vi "Periodic Tasks.vi"(8 "error out":errorcluster) -> ()   [LabVIEW 2011]
doc: "This VI runs in parallel to other tasks. It can contain as many user-defined periodic loops as you need. These can carry out PID or other sorts of timed response."
uses:
  <vilib>/Rock Robotics/WPI/Camera/WPI_CameraFrameRate.ctl
  <vilib>/Rock Robotics/WPI/Camera/WPI_CameraImageSize.ctl
  <vilib>/Rock Robotics/SystemInterfaces/DIO/FPGA_DIOChannel.ctl
  <vilib>/Rock Robotics/SystemInterfaces/Typedef/FPGA_TypedefDigitalModule.ctl
  <vilib>/Rock Robotics/WPI/Relay/WPI_RelayValue.ctl
  <vilib>/Rock Robotics/WPI/Counter/WPI_CounterDigitalInputToDigitalSource.vi
  Robot Global Data.vi
panel:
  out "Lights?":bool
  in  "Density Threshold":dbl=3.0
  in  "Dense Adjustment Factor":dbl=0.89
  out "Pressure":dbl
  out "Integral":dbl
  out "Error":dbl
  out "Waveform Chart":dynamicdata(graph)
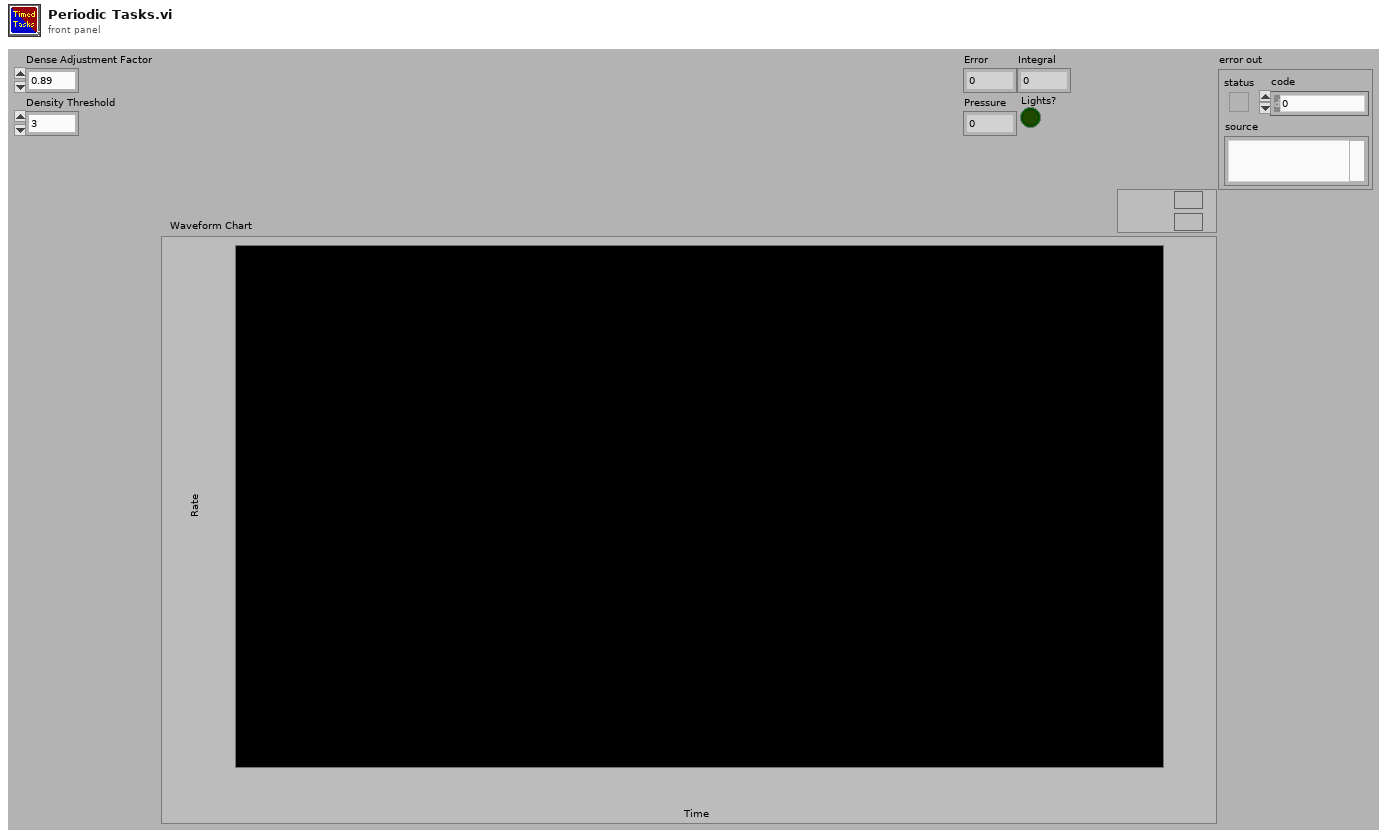
[diagram p1: front panel]
types:
  T1 = typedef "FPGA_DIOChannel.ctl" = enum8{"DIO 1", "DIO 2", "DIO 3", "DIO 4", "DIO 5", "DIO 6", "DIO 7", "DIO 8", "DIO 9", "DIO 10", "DIO 11", "DIO 12", "DIO 13", "DIO 14", "Invalid"}
  T2 = typedef "FPGA_TypedefDigitalModule.ctl" = enum16{"Digital Module 1", "Digital Module 2"}
  T3 = typedef "WPI_CameraImageSize.ctl" = enum16{"640x480", "320x240", "160x120"}
  T4 = typedef "WPI_CameraFrameRate.ctl" = u32
  T5 = typedef "WPI_JoystickDevRef.ctl" = cluster{"Device":T6}
  T6 = typedef "WPI_JoystickDeviceEnum.ctl" = enum16{"USB 1", "USB 2", "USB 3", "USB 4", "Kinect 1", "Kinect 2"}
  T7 = typedef "WPI_JoystickButtonState.ctl" = cluster{"Button 1":bool, "Button 2":bool, "Button 3":bool, "Button 4":bool, "Button 5":bool, "Button 6":bool, "Button 7":bool, "Button 8":bool, "Button 9":bool, "Button 10":bool, "Button 11":bool, "Button 12":bool}
  T8 = typedef "WPI_CameraDevRef.ctl" = cluster{"Camera Address":string, "CameraStatus":errorcluster, "Acquire Image Notifier":refnum<notifier>}
  T9 = typedef "WPI_AnalogChannelDevRef.ctl" = cluster{"DevStatus":errorcluster, "Analog Module":T10, "Analog Channel":T11}
  T10 = typedef "FPGA_TypedefAnalogModule.ctl" = enum16{"Analog Module 1", "Analog Module 2"}
  T11 = typedef "FPGA_AIChannel.ctl" = enum8{"AI 1", "AI 2", "AI 3", "AI 4", "AI 5", "AI 6", "AI 7", "AI 8", "Invalid"}
  T12 = typedef "WPI_RelayValue.ctl" = enum16{"Off", "On", "Forward", "Reverse"}
  T13 = typedef "WPI_RelayDevRef.ctl" = cluster{"DevStatus":errorcluster, "Relay Channel":T14, "Digital Module":T2, "Relay Direction":T15}
  T14 = typedef "FPGA_DIORelayChannel.ctl" = enum8{"Relay 1", "Relay 2", "Relay 3", "Relay 4", "Relay 5", "Relay 6", "Relay 7", "Relay 8", "Invalid"}
  T15 = typedef "WPI_RelayDirection.ctl" = enum16{"Both directions", "Forward only", "Reverse only"}
  T16 = typedef "WPI_DigitalInputDevRef.ctl" = cluster{"DevStatus":errorcluster, "DIO Channel":T1, "Digital Module":T2}
  T17 = typedef "FPGA_CounterEncoderSourceConvertionLVSourceType.ctl" = cluster{"DevStatus":errorcluster, "AnalogTriggerMode?":bool, "DigitalMode":cluster{"Digital Module":T2, "DIO Channel":T18}, "AnalogTriggerMode":cluster{"AnalogTriggerIndex":T19, "OutputType":T20}}
  T18 = typedef "FPGA_DIODigitalSourceChannel.ctl" = enum8{"DIO 1", "DIO 2", "DIO 3", "DIO 4", "DIO 5", "DIO 6", "DIO 7", "DIO 8", "DIO 9", "DIO 10", "DIO 11", "DIO 12", "DIO 13", "DIO 14", "Disabled"}
  T19 = typedef "FPGA_AnalogTriggerIndex.ctl" = enum8{"Trig 0", "Trig 1", "Trig 2", "Trig 3", "Trig 4", "Trig 5", "Trig 6", "Trig 7", "Invalid"}
  T20 = typedef "FPGA_AnalogTriggerOutType.ctl" = enum16{"InWindow", "TriggerState", "Rising", "Falling"}
  T21 = typedef "WPI_EncoderDevRef.ctl" = cluster{"DevStatus":errorcluster, "EncoderIndex":T22, "CounterIndex":T23, "DistancePerCount":dbl, "Decoding Type":T24}
  T22 = typedef "FPGA_EncoderIdx.ctl" = enum8{"Enc 0", "Enc 1", "Enc 2", "Enc 3", "Invalid"}
  T23 = typedef "FPGA_CounterCtrSystemIndex.ctl" = enum8{"Ctr 0", "Ctr 1", "Ctr 2", "Ctr 3", "Ctr 4", "Ctr 5", "Ctr 6", "Ctr 7", "Invalid"}
  T24 = typedef "WPI_EncoderType.ctl" = enum16{"1x", "2x", "4x"}
  T25 = typedef "WPI_MotorControlDeviceRef.ctl" = cluster{"DeviceStatus":errorcluster, "Type":enum16{"PWM", "CAN"}, "PWM":cluster{"Digital Module":T2, "PWM Channel":T26, "DeadBand":T27}, "CAN":cluster{"Device Number":u8, "Control Mode":T28, "Semaphore":T29, "Max Vout":dbl}, "Invert":bool, "TransformRef":T30, "InvTransformRef":T30}
  T26 = typedef "FPGA_DIOPWMChannel.ctl" = enum8{"PWM 1", "PWM 2", "PWM 3", "PWM 4", "PWM 5", "PWM 6", "PWM 7", "PWM 8", "PWM 9", "PWM 10", "Invalid"}
  T27 = typedef "WPI_PWMDeadband.ctl" = cluster{"Name":string, "maxPositivePwm":i32, "minPositivePwm":i32, "centerPwm":i32, "maxNegativePwm":i32, "minNegativePwm":i32, "angularRange":u16}
  T28 = typedef "WPI_CANJaguar_ControlMode.ctl" = enum8{"Percent VBus", "Current", "Speed", "Position", "Voltage"}
  T29 = typedef "Semaphore RefNum" = refnum<k1>
  T30 = typedef "WPI_PWMTransform_ConPane.ctl" = refnum<vi>
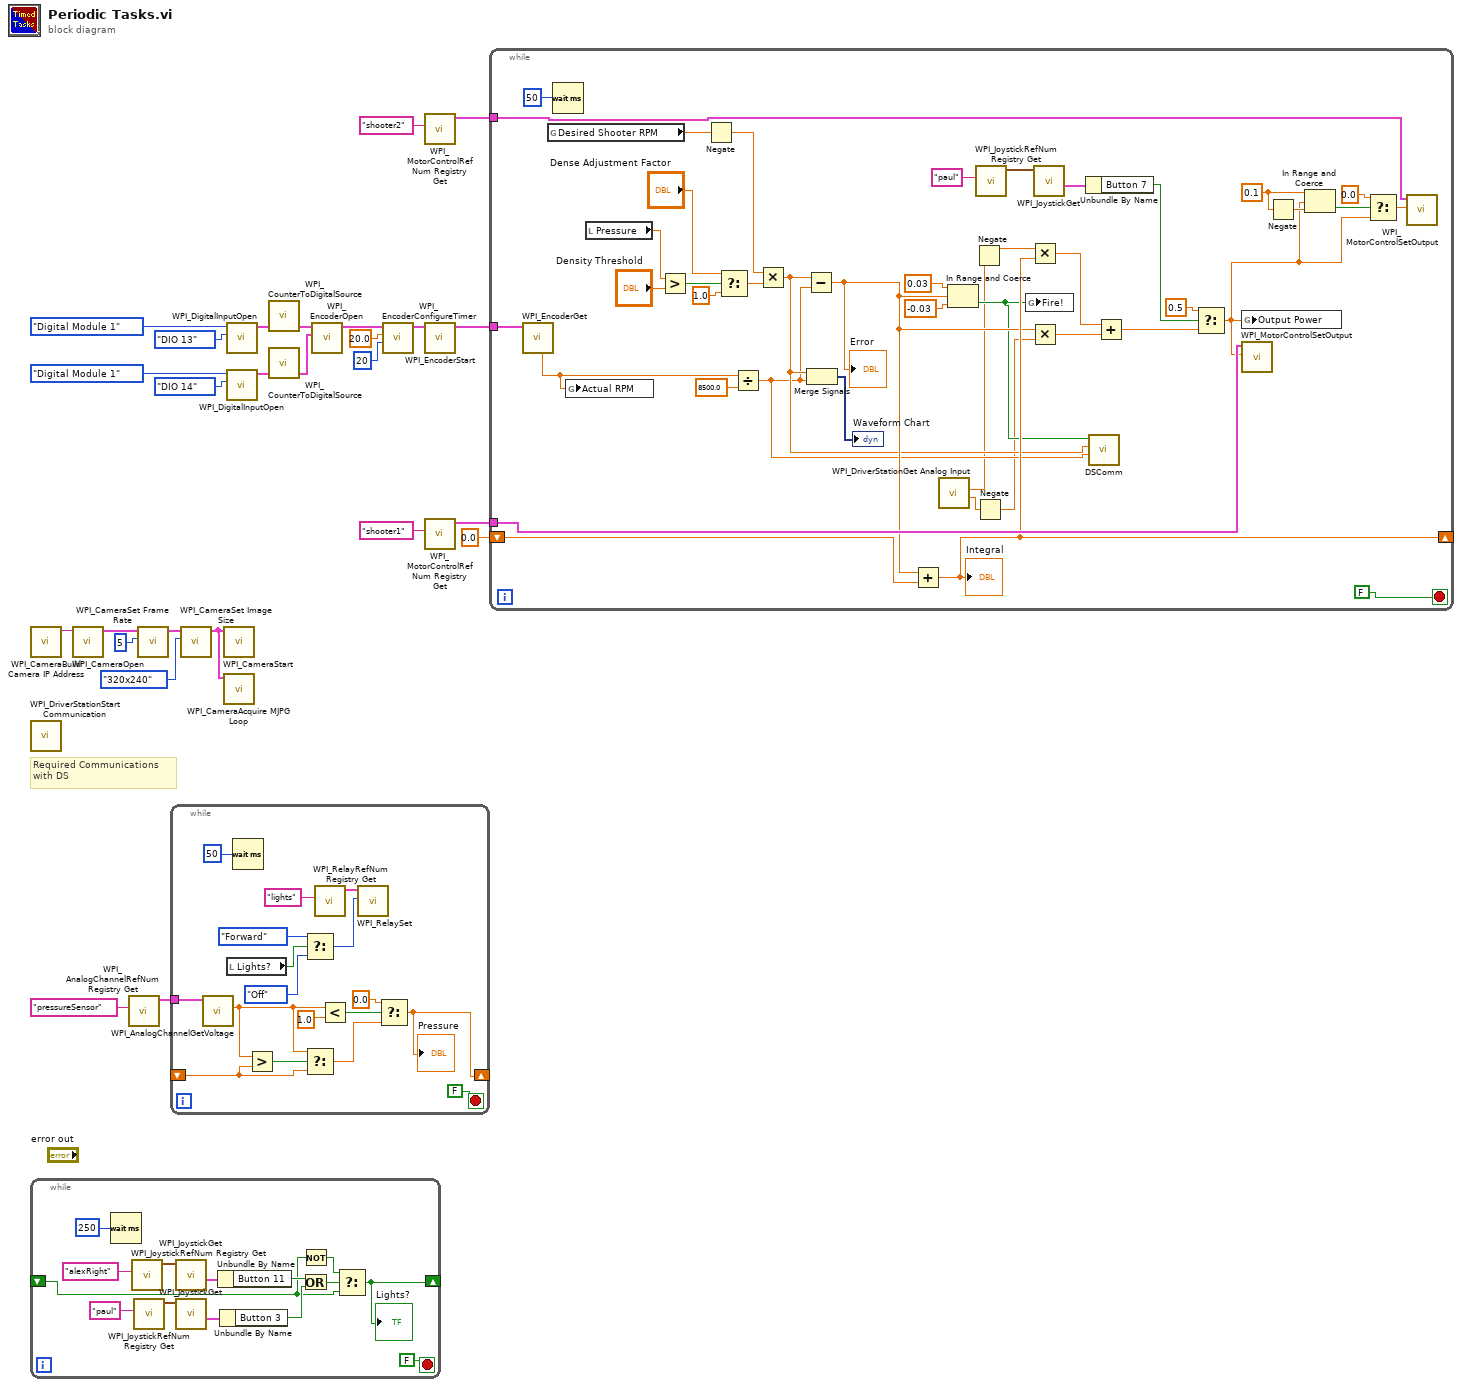
[diagram p0: block diagram]
diagram:
  # "Required Communications\nwith DS"
  n1 = call <vilib>:"WPI_CameraBuild Camera IP Address.vi"() -> ("Camera Address"=w22:string)  [unwired: 11 in]
  n2 = call <vilib>:"WPI_DriverStationStart Communication.vi"() -> ()  [unwired: 1 in, 11 out]
  n3 = while {
    shift-right: [w30] -> _
    shift-left: _ -> [w29]
    stop <- FALSE stop-if-true
    n4 = Wait (ms)(milliseconds to wait=u32 250) -> ()  [unwired: 1 out]
    n5 = call <vilib>:"WPI_JoystickRefNum Registry Get.vi"("refnum name"="alexRight") -> ("JoystickDevRef"=w38:T5)  [unwired: 9 in, 1 out]
    n6 = call <vilib>:"WPI_JoystickRefNum Registry Get.vi"("refnum name"="paul") -> ("JoystickDevRef"=w37:T5)  [unwired: 9 in, 1 out]
    n7 = call <vilib>:"WPI_JoystickGet.vi"("JoystickDevRef"=w38) -> ("Buttons"=w40:T7)  [unwired: 4 in, 2 out]
    n8 = call <vilib>:"WPI_JoystickGet.vi"("JoystickDevRef"=w37) -> ("Buttons"=w35:T7)  [unwired: 4 in, 2 out]
    n9 = Unbundle By Name(w40) -> ("Button 11"=w34:bool)
    n10 = Unbundle By Name(w35) -> ("Button 3"=w33:bool)
    n11 = Not(x=w29) -> (.not. x?=w31:bool)
    n12 = Or(x=w34, y=w33) -> (x .or. y?=w32:bool)
    n13 = Select(t=w31, s=w32, f=w29) -> (s? t:f=w30:bool)
    "Lights?" <- w30
  }
  n14 = call <vilib>:"WPI_CameraOpen.vi"("Camera Address"=w22) -> ("CameraDevRef"=w24:T8)  [unwired: 1 in, 9 out]
  n15 = call <vilib>:"WPI_AnalogChannelRefNum Registry Get.vi"("refnum name"="pressureSensor") -> ("AIDeviceRef"=w1:T9)  [unwired: 9 in, 1 out]
  n16 = call <vilib>:"WPI_CameraSet Frame Rate.vi"("Frame Rate (fps)"=T4 5, "CameraDevRef"=w24) -> ("CameraDevRef Out"=w25:T8)  [unwired: 1 in, 8 out]
  n17 = while {
    tunnel: w1 -> [w56]
    shift-right: [w48] -> _
    shift-left: _ -> [w54]
    stop <- FALSE stop-if-true
    n18 = call <vilib>:"WPI_AnalogChannelGetVoltage.vi"("AIDeviceRef"=w56) -> ("Voltage"=w52:dbl)  [unwired: 8 in, 2 out]
    n19 = local read "Lights?"() -> (w45:bool)
    n20 = Wait (ms)(milliseconds to wait=u32 50) -> ()  [unwired: 1 out]
    n21 = Greater?(x=w52, y=w54) -> (0:w55:bool)
    n22 = Select(t=WPI_RelayValue."Forward" ("RelayValue"), s=w45, f=WPI_RelayValue."Off" ("RelayValue")) -> (s? t:f=w43:T12)
    n23 = Select(t=w52, s=w55, f=w54) -> (s? t:f=w53:dbl)
    n24 = call <vilib>:"WPI_RelayRefNum Registry Get.vi"("refnum name"="lights") -> ("RelayDevRef"=w41:T13)  [unwired: 9 in, 1 out]
    n25 = Less?(x=w52, y=1.0) -> (x < y?=w50:bool)
    n26 = call <vilib>:"WPI_RelaySet.vi"("RelayValue"=w43, "RelayDevRef"=w41) -> ()  [unwired: 8 in, 2 out]
    n27 = Select(t=0.0, s=w50, f=w53) -> (s? t:f=w48:dbl)
    "Pressure" <- w48
  }
  n28 = call <vilib>:"WPI_CameraSet Image Size.vi"("Image Size"=WPI_CameraImageSize."320x240", "CameraDevRef"=w25) -> ("CameraDevRef Out"=w21:T8)  [unwired: 1 in, 8 out]
  n29 = call <vilib>:"WPI_CameraStart.vi"("CameraDevRef"=w21) -> ()  [unwired: 1 in, 10 out]
  n30 = call <vilib>:"WPI_CameraAcquire MJPG Loop.vi"("CameraDevRef"=w21) -> ()  [unwired: 11 in]
  n31 = call <vilib>:"WPI_DigitalInputOpen.vi"("DIO Channel"=FPGA_DIOChannel."DIO 13", "Digital Module (Module 1)"=FPGA_TypedefDigitalModule."Digital Module 1") -> ("DigitalInputDevRef"=w13:T16)  [unwired: 1 in, 8 out]
  n32 = call <vilib>:"WPI_DigitalInputOpen.vi"("DIO Channel"=FPGA_DIOChannel."DIO 14", "Digital Module (Module 1)"=FPGA_TypedefDigitalModule."Digital Module 1") -> ("DigitalInputDevRef"=w12:T16)  [unwired: 1 in, 8 out]
  n33 = call-poly <vilib>:"WPI_CounterToDigitalSource.vi"("DigitalInputDevRef"=w13) -> ("Digital Source"=w11:T17)  [unwired: 6 out]
  n34 = call-poly <vilib>:"WPI_CounterToDigitalSource.vi"("DigitalInputDevRef"=w12) -> ("Digital Source"=w10:T17)  [unwired: 6 out]
  n35 = call <vilib>:"WPI_EncoderOpen.vi"("BSource"=w10, "ASource"=w11) -> ("EncoderDevRef"=w14:T21)  [unwired: 6 in, 3 out]
  n36 = call <vilib>:"WPI_EncoderConfigureTimer.vi"("Number Samples to Average"=u8 20, "Minimum Rate"=20.0, "EncoderDevRef"=w14) -> ("EncoderDevRef"=w16:T21)  [unwired: 1 in, 7 out]
  n37 = call <vilib>:"WPI_MotorControlRefNum Registry Get.vi"("refnum name"="shooter2") -> ("MotorControlDevRef"=w18:T25)  [unwired: 9 in, 1 out]
  n38 = call <vilib>:"WPI_EncoderStart.vi"("EncoderDevRef"=w16) -> ("EncoderDevRef"=w15:T21)  [unwired: 1 in, 9 out]
  n39 = call <vilib>:"WPI_MotorControlRefNum Registry Get.vi"("refnum name"="shooter1") -> ("MotorControlDevRef"=w17:T25)  [unwired: 9 in, 1 out]
  n40 = while {
    tunnel: w18 -> [w98]
    tunnel: w17 -> [w97]
    shift-right: [w93] -> _
    shift-left: 0.0 -> [w94]
    tunnel: w15 -> [w92]
    stop <- FALSE stop-if-true
    w69 = 0.1 ("upper limit")
    n41 = call <vilib>:"WPI_EncoderGet.vi"("EncoderDevRef"=w92) -> ("Rate"=w72:dbl)  [unwired: 5 in, 5 out]
    n42 = global read "Robot Global Data.vi" "Desired Shooter RPM"() -> (w90:dbl)
    n43 = Wait (ms)(milliseconds to wait=u32 50) -> ()  [unwired: 1 out]
    n44 = global write "Robot Global Data.vi" "Actual RPM"(w72) -> ()
    n45 = local read "Pressure"() -> (w87:dbl)
    n46 = Greater?(x=w87, y="Density Threshold") -> (0:w84:bool)
    n47 = Negate(x=w90) -> (-x=w91:dbl)
    n48 = Select(t="Dense Adjustment Factor", s=w84, f=1.0) -> (s? t:f=w85:dbl)
    n49 = Divide(x=w72, y=8500.0) -> (x/y=w62:dbl)
    n50 = Multiply(x=w91, y=w85) -> (x*y=w63:dbl)
    n51 = Subtract(x=w63, y=w62) -> (x-y=w75:dbl)
    "Error" <- w75
    n52 = Merge Signals(w63, w62) -> (→"Waveform Chart":dynamicdata)
    n53 = Add(x=w75, y=w94) -> (x+y=w93:dbl)
    "Integral" <- w93
    n54 = call <vilib>:"WPI_DriverStationGet Analog Input.vi"() -> ("Analog 3 (V)"=w58:dbl, "Analog 2 (V)"=w61:dbl)  [unwired: 10 out]
    n55 = In Range and Coerce(upper limit=0.03, x=w75, lower limit=-0.03) -> (In Range?=w64:bool)  [unwired: 1 out]
    n56 = Negate(x=w61) -> (-x=w60:dbl)
    n57 = Negate(x=w58) -> (-x=w59:dbl)
    n58 = call <vilib>:"WPI_JoystickRefNum Registry Get.vi"("refnum name"="paul") -> ("JoystickDevRef"=w80:T5)  [unwired: 9 in, 1 out]
    n59 = global write "Robot Global Data.vi" "Fire!"(w64) -> ()
    n60 = Multiply(x=w60, y=w93) -> (x*y=w76:dbl)
    n61 = Multiply(x=w75, y=w59) -> (x*y=w74:dbl)
    n62 = call <vilib>:"WPI_JoystickGet.vi"("JoystickDevRef"=w80) -> ("Buttons"=w79:T7)  [unwired: 4 in, 2 out]
    n63 = Unbundle By Name(w79) -> ("Button 7"=w78:bool)
    n64 = call "DSComm.vi"("Actual RPM"=w62, "Desired RPM"=w63, "Fire?"=w64) -> ()  [unwired: 8 in, 1 out]
    n65 = Add(x=w76, y=w74) -> (x+y=w73:dbl)
    n66 = Select(t=0.5, s=w78, f=w73) -> (s? t:f=w66:dbl)
    n67 = global write "Robot Global Data.vi" "Output Power"(w66) -> ()
    n68 = call <vilib>:"WPI_MotorControlSetOutput.vi"("Output"=w66, "MotorControlDevRef"=w97) -> ()  [unwired: 8 in, 2 out]
    n69 = Negate(x=w69) -> (-x=w68:dbl)
    n70 = In Range and Coerce(upper limit=w69, x=w66, lower limit=w68) -> (In Range?=w70:bool)  [unwired: 1 out]
    n71 = Select(t=0.0, s=w70, f=w66) -> (s? t:f=w65:dbl)
    n72 = call <vilib>:"WPI_MotorControlSetOutput.vi"("Output"=w65, "MotorControlDevRef"=w98) -> ()  [unwired: 8 in, 2 out]
  }
